vi "FFT Co-processor (Host)-1.vi"() -> ()   [LabVIEW 2015]
doc: "Uses the FPGA target as a co-processor that continuously computes the FFT of the user controlled signal.\n\nThe three signal are generated, added together, and sent through a DMA FIFO to the FPGA target. The data is then placed in a target-scoped FIFO and sent to the FFT Express VI, where the FFT of the data is computed. The FFT signal is then placed in a target-scoped FIFO and written back to the host through a DMA FIFO. The resulting FFT data is scaled and displayed on the host front panel."
uses:
  <vilib>/rvi/interface/nirviOpenFPGA/nirviOpenFPGA.xnode
  <vilib>/rvi/interface/nirviMethod/nirviMethod.xnode
  <vilib>/rvi/interface/nirviCloseFPGA/nirviCloseFPGA.xnode
  Fpga-Version/PXI-7953R/FFT Co-processor (FPGA).vi
  <vilib>/rvi/errors/niLvFpgaMergeErrorWithErrorCode.vi
panel:
  out "Data Sent In.size":i32
  out "Data Sent In":csg[](array[numeric])
  out "Fft Out (2)":csg[](array[numeric])
  out "Error":csg[](array[numeric])
  out "FFT Out":csg[](array[numeric])
  out "Receiving Loop":i32
  in  "Expected FFT {X}":csg[](array[numeric]) format="%.7g"
  in  "Chirped Data":csg[](array[numeric])=[0.0+1.0i, 1.0+2.0i, 3.0+0.55i, 0.0+0.0i, 0.0+1.0i, 1.0+2.0i, 3.0+0.55i, 0.0+0.0i]
  out "data out":i32
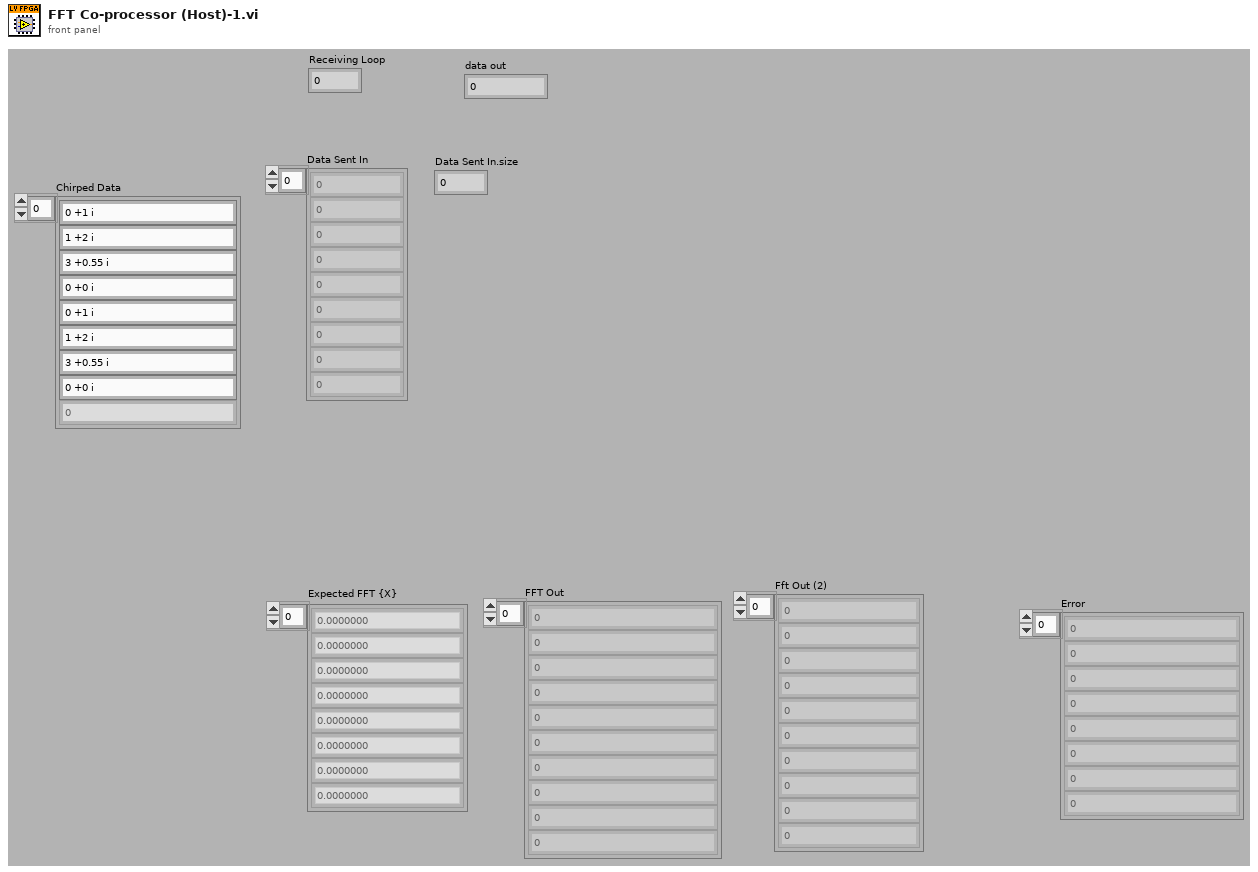
[diagram p1: front panel]
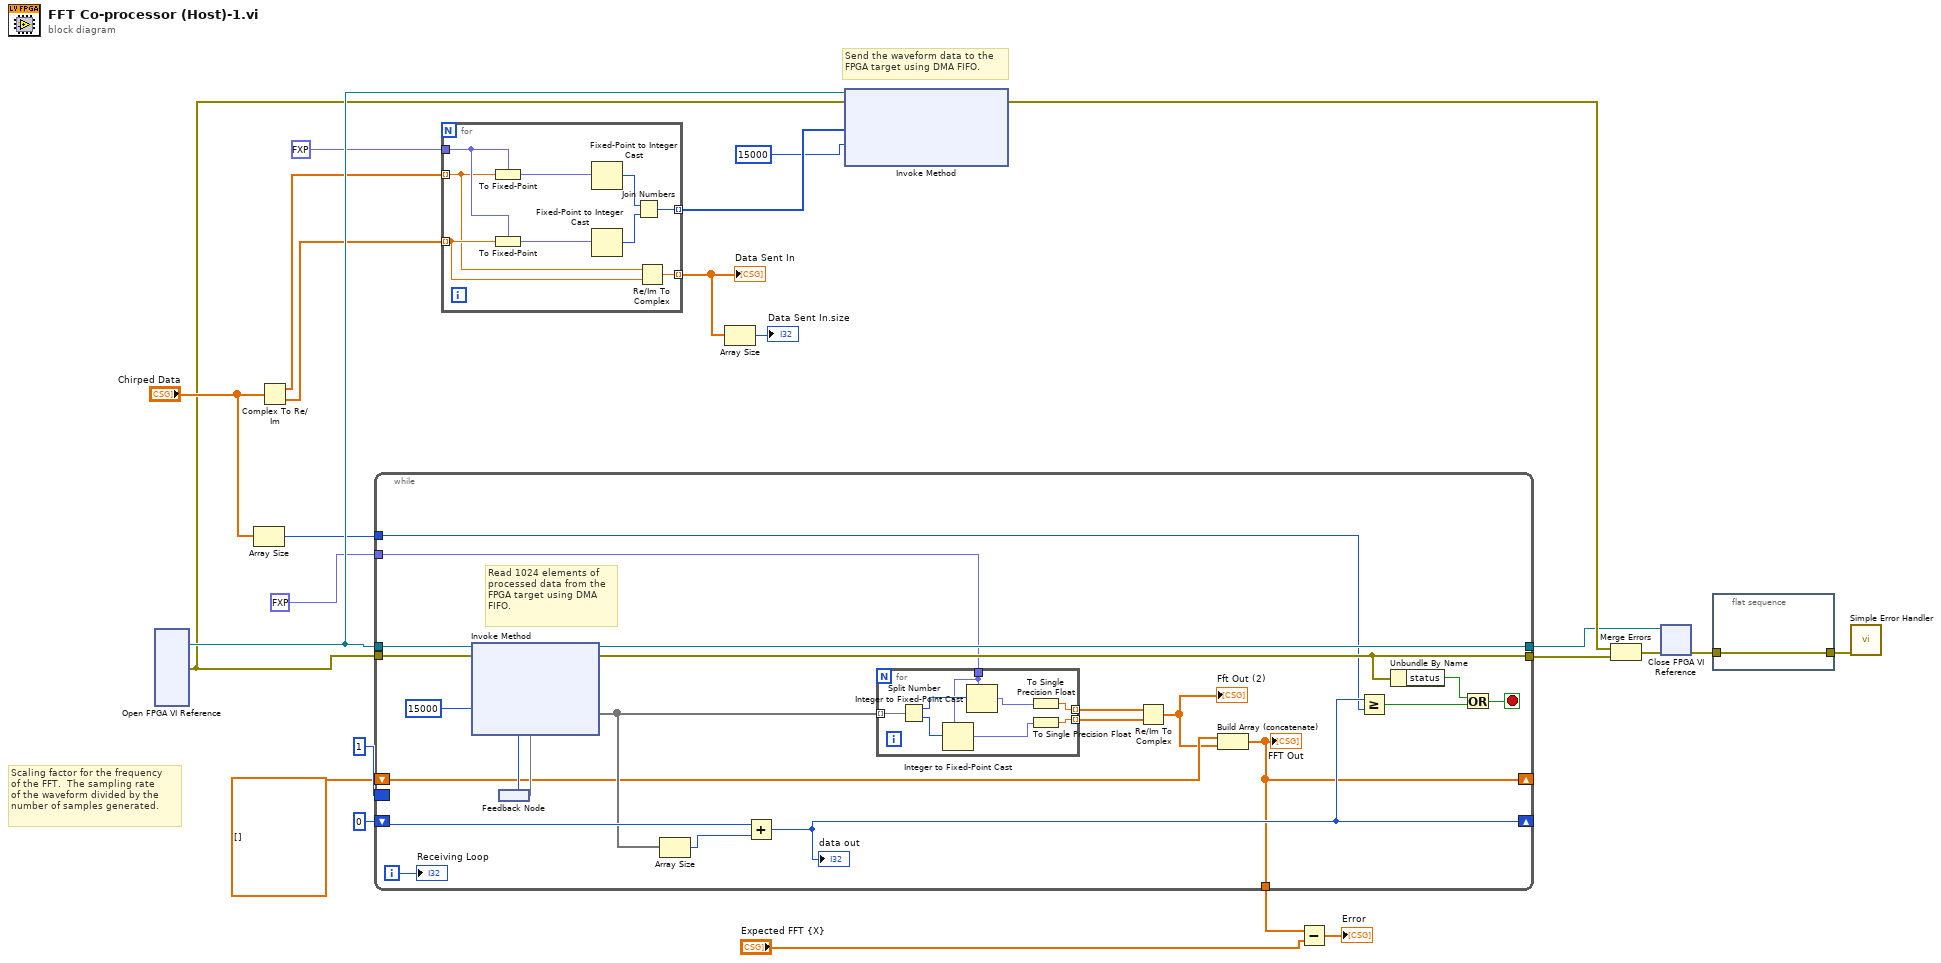
[diagram p0: block diagram]
diagram:
  # "Send the waveform data to the\nFPGA target using DMA FIFO."
  # "Scaling factor for the frequency \nof the FFT.  The sampling rate \nof the waveform divided by the \nnumber of samples generated."
  n1 = xnode "Open FPGA VI Reference"() -> ("FPGA VI Reference Out"=w24:refnum<k20>, "error out"=w2:errorcluster)  [unwired: 2 in]
  n2 = Array Size(array="Chirped Data") -> (size(s)=w14:i32)
  n3 = Complex To Re/Im(x + iy="Chirped Data") -> (x=w8:sgl[], y=w7:sgl[])
  n4 = while {
    tunnel: w24 -> [w45]
    tunnel: w2 -> [w44]
    tunnel: [w46] -> w20
    tunnel: [w42] -> w23
    shift-right: [w29] -> _
    shift-left: 0 -> [w41]
    border: u32 1 ("Elements Remaining") -> [_]
    shift-right: [w25] -> _
    shift-left: csg[] [] ("FFT Out") -> [w32]
    tunnel: w14 -> [w27]
    tunnel: fxp<+/-,28,8> 0.0 ("real data in") -> [w26]
    tunnel: [w25] -> w12
    i -> [w33]
    stop <- w43 stop-if-true
    # "Read 1024 elements of\nprocessed data from the\nFPGA target using DMA\nFIFO."
    n5 = feedback #1() -> (w34:u32)
    n6 = xnode "Invoke Method"("FPGA VI Reference In"=w45, "error in"=w44, "Number of Elements"=w34, "Timeout (ms)"=15000) -> ("FPGA VI Reference Out"=w46:refnum<k20>, "error out"=w42:errorcluster, "Data"=w40:void[], "Elements Remaining"=w35)
    n7 = feedback-in #1(w35) -> ()
    n8 = Array Size(array=w40) -> (size(s)=w39:i32)
    n9 = Add(x=w41, y=w39) -> (x+y=w29:i32)
    "data out" <- w29
    n10 = for {
      tunnel: w40 -> [w54] mode=indexing
      tunnel: [w53] -> w37 mode=indexing
      tunnel: [w52] -> w36 mode=indexing
      tunnel: w26 -> [w49]
      n11 = Split Number(x=w54) -> (hi(x)=w51:u16, lo(x)=w50:u16)
      n12 = Integer to Fixed-Point Cast(fixed-point type=w49, integer=w50) -> (fixed-point=w47:fxp<+/-,28,8>)
      n13 = Integer to Fixed-Point Cast(fixed-point type=w49, integer=w51) -> (fixed-point=w48:fxp<+/-,28,8>)
      n14 = To Single Precision Float(number=w48) -> (single precision float=w53:sgl)
      n15 = To Single Precision Float(number=w47) -> (single precision float=w52:sgl)
    }
    n16 = Re/Im To Complex(1:w36, 2:w37) -> (0:w31:csg[])
    "Fft Out (2)" <- w31
    n17 = Build Array (concatenate)(w32, w31) -> (w25:csg[])
    "FFT Out" <- w25
    n18 = Greater Or Equal?(x=w29, y=w27) -> (x >= y?=w30:bool)
    n19 = Unbundle By Name(w42) -> ("status"=w28:bool)
    n20 = Or(x=w28, y=w30) -> (x .or. y?=w43:bool)
    "Receiving Loop" <- w33
  }
  n21 = for {
    tunnel: w8 -> [w57] mode=indexing
    tunnel: w7 -> [w58] mode=indexing
    tunnel: [w60] -> w6 mode=indexing
    tunnel: fxp<+/-,24,4> 0.0 ("real data in") -> [w59]
    tunnel: [w56] -> w4 mode=indexing
    n22 = To Fixed-Point(fixed-point type=w59, number=w57) -> (fixed-point=w55:fxp<+/-,24,4>)
    n23 = To Fixed-Point(fixed-point type=w59, number=w58) -> (fixed-point=w62:fxp<+/-,24,4>)
    n24 = Fixed-Point to Integer Cast(1:w55) -> (0:w63:i32)
    n25 = Fixed-Point to Integer Cast(1:w62) -> (0:w61:i32)
    n26 = Join Numbers(hi=w63, lo=w61) -> ((hi.lo)=w60:u64)
    n27 = Re/Im To Complex(1:w58, 2:w57) -> (0:w56:csg)
  }
  "Data Sent In" <- w4
  n28 = Array Size(array=w4) -> (size(s)=→"Data Sent In.size":i32)
  n29 = xnode "Invoke Method"("FPGA VI Reference In"=w24, "error in"=w2, "Data"=w6, "Timeout (ms)"=15000) -> ("error out"=w22:errorcluster)  [unwired: 2 out]
  n30 = Subtract(x=w12, y="Expected FFT {X}") -> (x-y=→"Error":csg[])
  n31 = Merge Errors(w22, w23) -> (w21:errorcluster)
  n32 = xnode "Close FPGA VI Reference"("FPGA VI Reference In"=w20, "error in"=w21) -> ("error out"=w19:errorcluster)
  n33 = flat-sequence {
    tunnel: w19 -> [w64]
    tunnel: [w64] -> w18
    frame #0 {
    }
  }
  n34 = call <vilib>:"Simple Error Handler.vi"("error in (no error)"=w18) -> ()  [unwired: 1 in, 8 out]
